vi "Close Command.vi"(0 "SLSC Remote in":refnum<class "SLSC Remote.lvclass">, 5 "command":refnum<k21>, 11 "error in (no error)":errorcluster) -> (4 "SLSC Remote out":refnum<class "SLSC Remote.lvclass">, 15 "error out":errorcluster)   [LabVIEW 2016, in "SLSC Interfaces.lvlib" / "SLSC Remote.lvclass"]
uses:
  SLSC Remote.lvclass
  <vilib>/NI/NI JSONRPC Server Framework/Classes/Server/JSONRPC Server.lvclass
  <vilib>/httpClient/LabVIEWHTTPClient.lvlib
  <vilib>/httpClient/POSTBuffer.vi
  <vilib>/NI/JSON Support for LabVIEW/JSON Data Classes/JSON Helper/JSON Helper.lvclass
  <vilib>/NI/JSON Support for LabVIEW/JSON Data Classes/JSON Object/New JSON Object (Single String).vi
  <vilib>/NI/JSON Support for LabVIEW/JSON Data Classes/JSON Object/JSON Object.lvclass
  <vilib>/NI/NI JSONRPC Server Framework/Classes/Server/Format Client Request (Auto-Increment).vi
  <vilib>/NI/NI JSONRPC Server Framework/Classes/Server/Parse Response (Object).vi
  C:/Program Files (x86)/National Instruments/LabVIEW 2016/vi.lib/NI/JSON Support for LabVIEW/JSON Data Classes/JSON Structured Type/JSON Structure.lvclass
  C:/Program Files (x86)/National Instruments/LabVIEW 2016/vi.lib/NI/JSON Support for LabVIEW/JSON Data Classes/JSON Datatype/JSON Null.lvclass
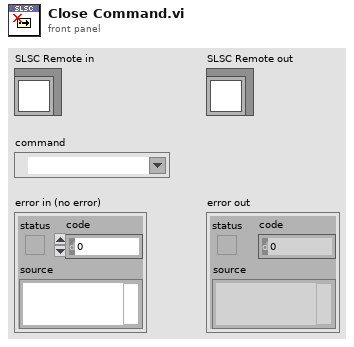
[diagram p1: front panel]
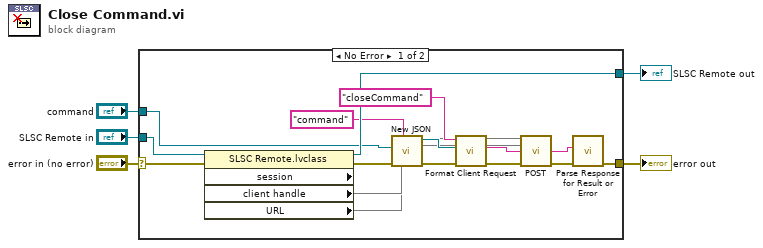
[diagram p0: block diagram]
diagram:
  n1 = case shown="No Error" "error in (no error)" {
    selector: "error in (no error)" -> [w18 w22]
    tunnel: "SLSC Remote in" -> [w20 w23]
    tunnel: [w19 w23] -> w4
    tunnel: [w8 w22] -> w3
    tunnel: "command" -> [w6 _]
    frame No Error {
      n2 = property class="SLSC Remote.lvclass" props=["session", "client handle", "URL"](reference=w20, error in=w18) -> (reference out=w19:refnum<class "SLSC Remote.lvclass">, error out=w17:errorcluster, "client handle"=w13, "URL"=w12)  [unwired: 1 out]
      n3 = call-poly <vilib>:"New JSON.vi"("key"="command" ("Name"), "error in (no error)"=w17, "value"=w6) -> ("error out"=w16:errorcluster, "JSON Object out"=w21:refnum<class "JSON Object.lvclass">)  [unwired: 7 in]
      n4 = call-poly <vilib>:"Format Client Request.vi"("error in (no error)"=w16, "JSON in"=w21, "method"="closeCommand") -> ("error out"=w11:errorcluster, "Request String"=w14:string)  [unwired: 7 in]
      n5 = call-poly <vilib>:"POST.vi"("client handle"=w13, "url"=w12, "buffer"=w14, "error in (no error)"=w11) -> ("body"=w10:string, "error out"=w9:errorcluster)  [unwired: 8 in, 2 out]
      n6 = call-poly <vilib>:"Parse Response for Result or Error.vi"("error in"=w9, "Response String In"=w10) -> ("error out"=w8:errorcluster)  [unwired: 7 in, 2 out]
    }
    frame Error {
    }
  }
  "error out" <- w3
  "SLSC Remote out" <- w4
